vi "KE622x -- Get Current Range tmp.vi"(0 "Resource In":refnum<visa-resource-name>, 1 "Check For SCPI Errors? (T)":bool=TRUE, 11 "error in (no error)":errorcluster) -> (4 "Resource Out (dupl)":refnum<visa-resource-name>, 8 "Current Range":T1, 15 "error out":errorcluster)   [LabVIEW 2016, in "Keithley 622x tmp.lvlib"]
doc: "Returns the state of auto-ranging and the selected range. Note that the selected range was selected by the instrument if auto-range is True, else it was previously specified by the user."
uses:
  Keithley 622x tmp.lvlib
  Typedefs/KE622x -- Current Range tmp.ctl
  Typedefs/KE622x -- Current Ranges tmp.ctl
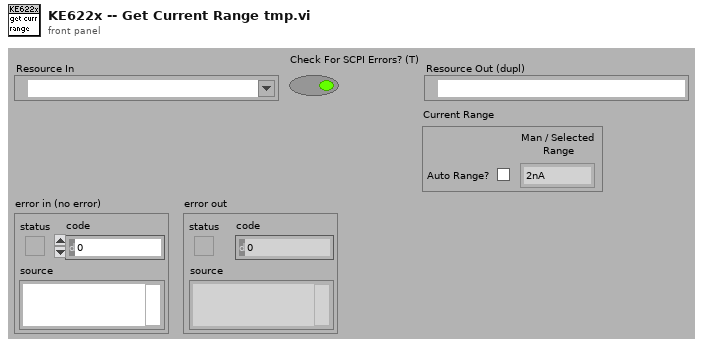
[diagram p1: front panel]
types:
  T1 = typedef "Keithley 622x tmp.lvlib/KE622x -- Current Range tmp.ctl" = cluster{"Auto Range?":bool, "Man / Selected\nRange":T2}
  T2 = typedef "Keithley 622x tmp.lvlib/KE622x -- Current Ranges tmp.ctl" = enum16{"2nA", "20nA", "200nA", "2uA", "20uA", "200uA", "2mA", "20mA", "100mA"}
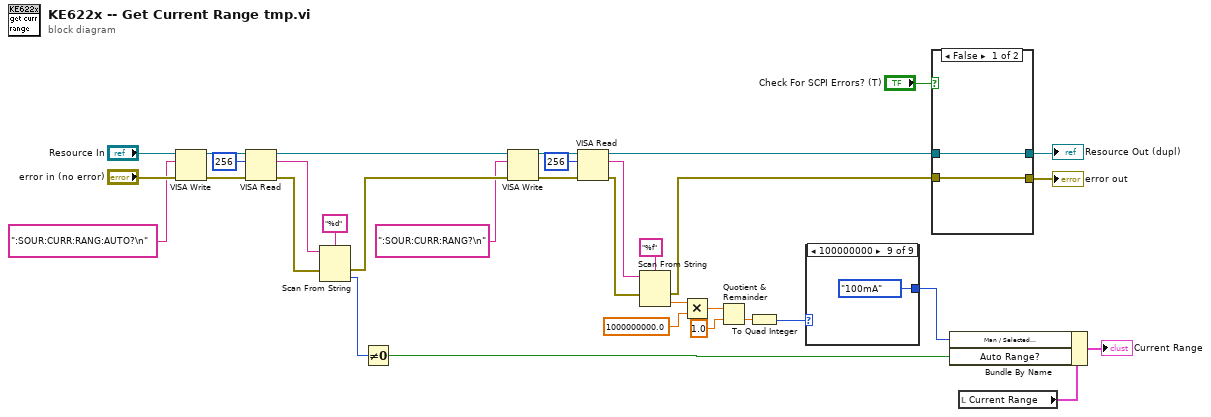
[diagram p0: block diagram]
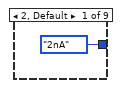
[diagram p2: hidden frame]
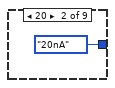
[diagram p3: hidden frame]
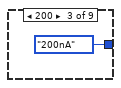
[diagram p4: hidden frame]
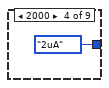
[diagram p5: hidden frame]
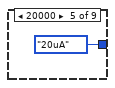
[diagram p6: hidden frame]
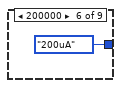
[diagram p7: hidden frame]
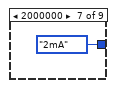
[diagram p8: hidden frame]
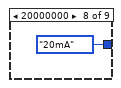
[diagram p9: hidden frame]
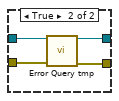
[diagram p10: hidden frame]
diagram:
  n1 = VISA Write(VISA resource name="Resource In", write buffer=":SOUR:CURR:RANG:AUTO?\n" ("format string"), error in (no error)="error in (no error)") -> (VISA resource name out=w28:refnum<visa-resource-name>, error out=w27:errorcluster)  [unwired: 1 out]
  n2 = VISA Read(VISA resource name=w28, byte count=u32 256, error in (no error)=w27) -> (VISA resource name out=w17:refnum<visa-resource-name>, read buffer=w23:string, error out=w25:errorcluster)  [unwired: 1 out]
  n3 = Scan From String(format string="%d", input string=w23, error in=w25) -> (error out=w18:errorcluster, output 1=w22:i32)  [unwired: 2 in, 2 out]
  n4 = Not Equal To 0?(x=w22) -> (x != 0?=w13:bool)
  n5 = VISA Write(VISA resource name=w17, write buffer=":SOUR:CURR:RANG?\n" ("format string"), error in (no error)=w18) -> (VISA resource name out=w21:refnum<visa-resource-name>, error out=w20:errorcluster)  [unwired: 1 out]
  n6 = VISA Read(VISA resource name=w21, byte count=u32 256, error in (no error)=w20) -> (VISA resource name out=w15:refnum<visa-resource-name>, read buffer=w11:string, error out=w2:errorcluster)  [unwired: 1 out]
  n7 = Scan From String(format string="%f", input string=w11, error in=w2) -> (error out=w1:errorcluster, output 1=w9:dbl)  [unwired: 2 in, 2 out]
  n8 = Multiply(x=w9, y=1000000000.0) -> (x*y=w7:dbl)
  n9 = Quotient & Remainder(x=w7, y=1.0) -> (floor(x/y)=w5:dbl)  [unwired: 1 out]
  n10 = To Quad Integer(1:w5) -> (0:w4:i64)
  n11 = case shown="100000000" w4 {
    tunnel: [KE622x_--_Current_Ranges_tmp."2nA" ("Man / Selected\nRange") KE622x_--_Current_Ranges_tmp."20nA" ("Man / Selected\nRange") KE622x_--_Current_Ranges_tmp."200nA" ("Man / Selected\nRange") KE622x_--_Current_Ranges_tmp."2uA" ("Man / Selected\nRange") KE622x_--_Current_Ranges_tmp."20uA" ("Man / Selected\nRange") KE622x_--_Current_Ranges_tmp."200uA" ("Man / Selected\nRange") KE622x_--_Current_Ranges_tmp."2mA" ("Man / Selected\nRange") KE622x_--_Current_Ranges_tmp."20mA" ("Man / Selected\nRange") KE622x_--_Current_Ranges_tmp."100mA" ("Man / Selected\nRange")] -> w12
    frame 2, Default {
    }
    frame 20 {
    }
    frame 200 {
    }
    frame 2000 {
    }
    frame 20000 {
    }
    frame 200000 {
    }
    frame 2000000 {
    }
    frame 20000000 {
    }
    frame 100000000 {
    }
  }
  n12 = case shown="False" "Check For SCPI Errors? (T)" {
    tunnel: w15 -> [w45 w49]
    tunnel: w1 -> [w44 w48]
    tunnel: [w44 w47] -> w30
    tunnel: [w45 w46] -> w31
    frame False {
    }
    frame True {
      n13 = call "Error Query tmp.vi"("VISA Resource In"=w49, "error in (no error)"=w48) -> ("VISA Resource Out (dupl)"=w46:refnum<visa-resource-name>, "error out"=w47:errorcluster)  [unwired: 10 in, 2 out]
    }
  }
  "Resource Out (dupl)" <- w31
  "error out" <- w30
  n14 = local read "Current Range"() -> (w14:T1)
  n15 = Bundle By Name(cluster=w14, "Man / Selected\nRange"=w12, "Auto Range?"=w13) -> (→"Current Range":T1)
